vi "Save to Excel (SubVI).vi"(0 "File Path Input":path, 1 "Save (Enable/Signal)":bool, 2 "Save Interval (s)":dbl=1.0, 3 "Title Block Array":string[](array[string]), 4 "Column Header Array":string[](array[string]), 5 "Data Array (Row)":string[](array[string]), 7 "File Configuration":T1={"Row Limit"=65500, "Default File Name"="Data", "New File Daily?"=TRUE, "Manual Save Interval?"=FALSE}, 9 "Change Save Location?":bool, 11 "Reset Elapsed Time":bool caption="Reset Elapsed Time?", 13 "Comments":string) -> (14 "File Path Output":path, 15 "Save Indicator":bool, 16 "# of Rows Saved":i32, 17 "Elapsed Time":string="00:00:00", 19 "Error Output":errorcluster)   [LabVIEW 2009]
panel:
  # "SAVE TO EXCEL SUBVI\nSave 1D Array (Row) to File"
  # "Created by Blake Otting 3/7/2007\nLast Updated 4/8/2010"
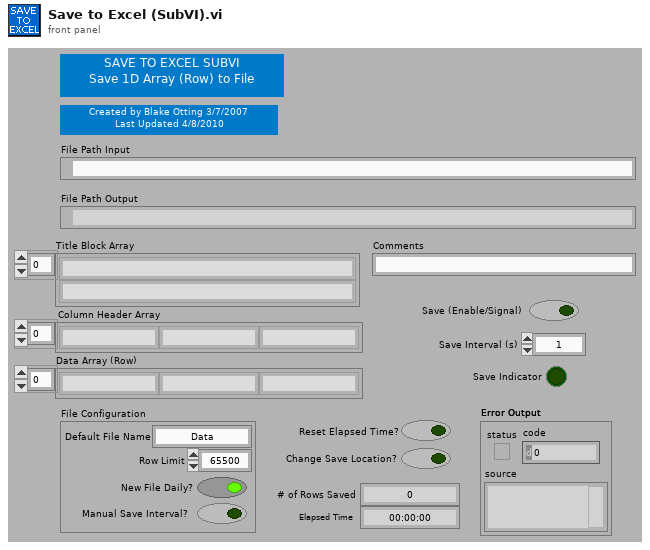
[diagram p1: front panel]
types:
  T1 = cluster{"Row Limit":i32, "Default File Name":string, "New File Daily?":bool, "Manual Save Interval?":bool}
  T2 = typedef "LVDateTimeRec.ctl" = cluster{"fractional second":dbl, "second":i32, "minute":i32, "hour":i32, "day of month":i32, "month":i32, "year":i32, "day of week":i32, "day of year":i32, "DST":i32}
  T3 = enum16{"open", "replace", "create", "open or create", "replace or create", "replace or create with confirmation"}
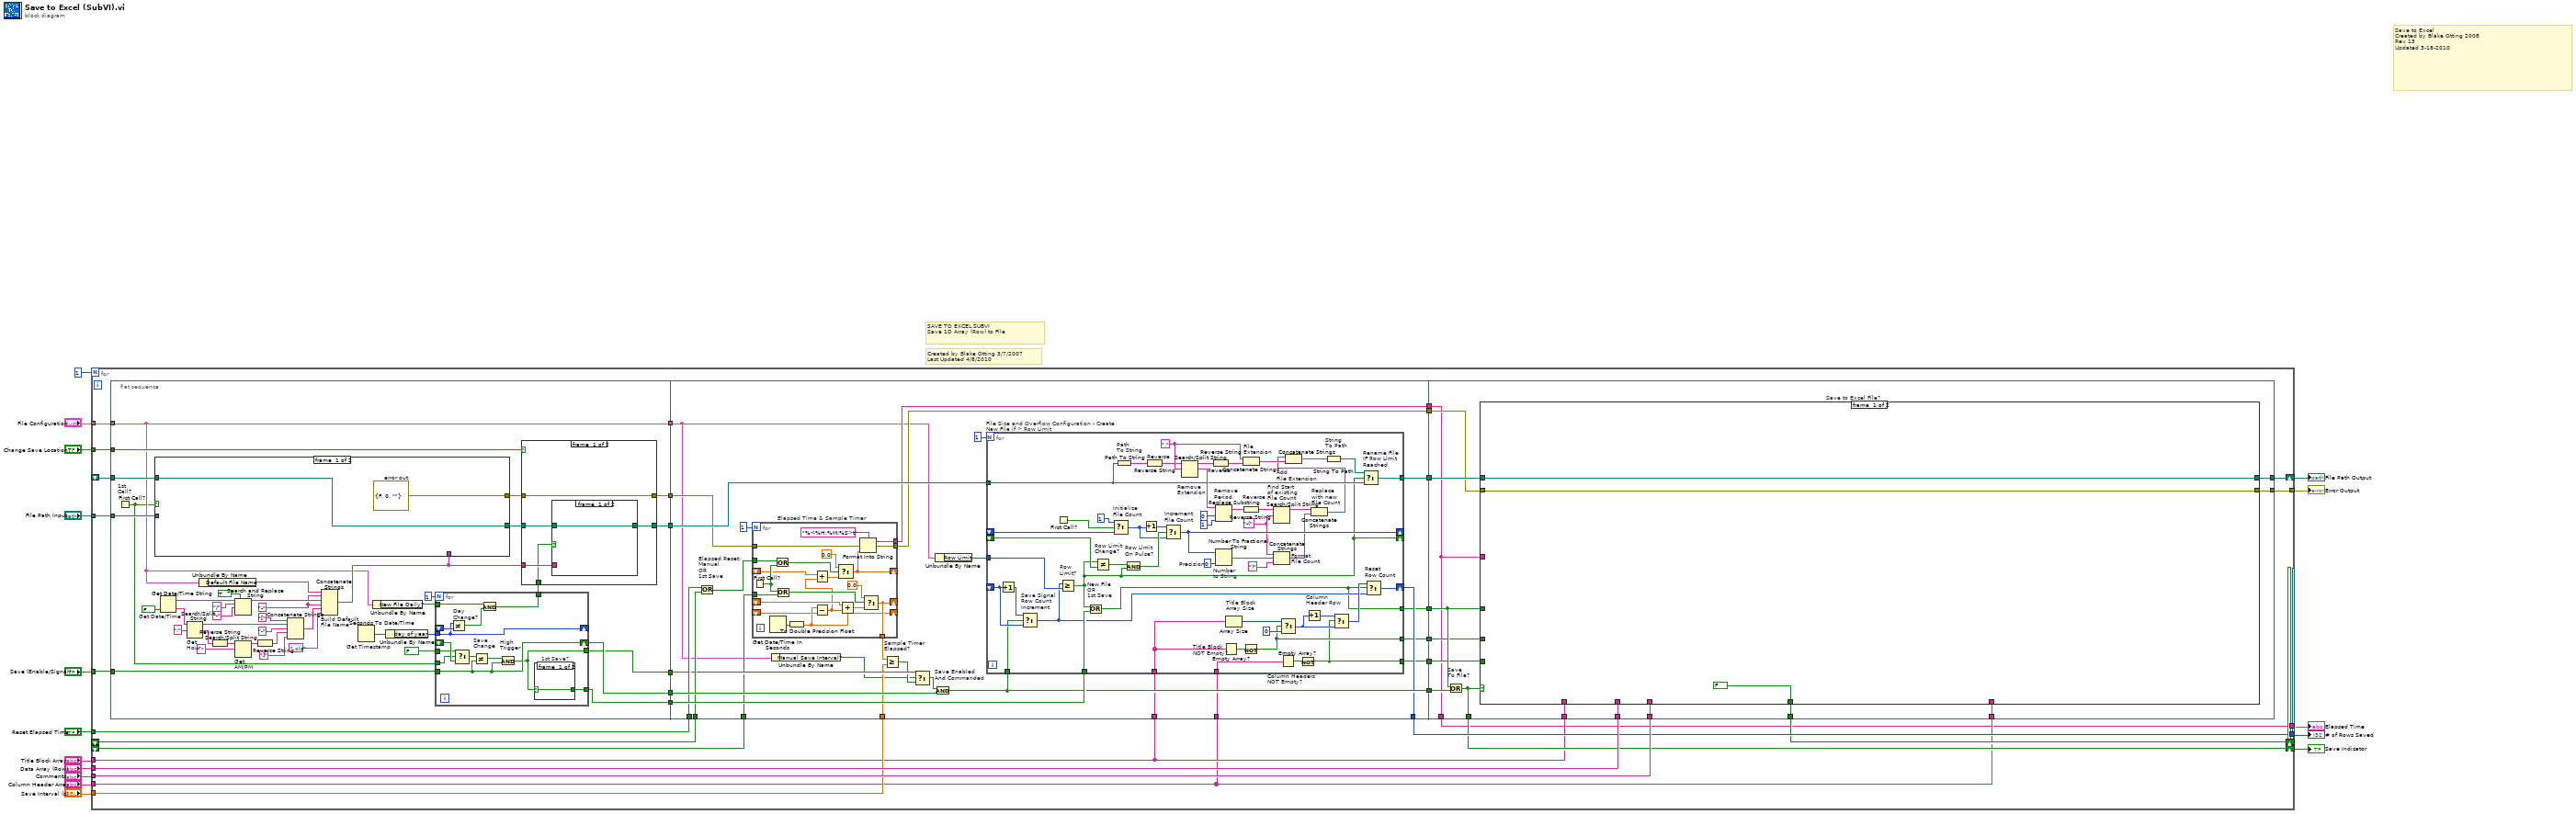
[diagram p0: block diagram]
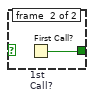
[diagram p2: hidden frame]
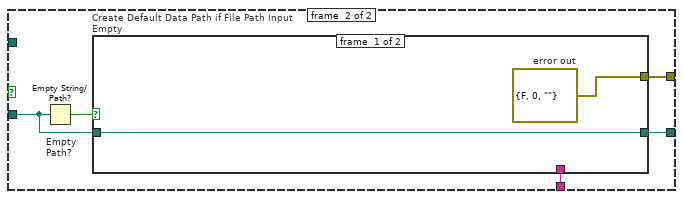
[diagram p3: hidden frame]
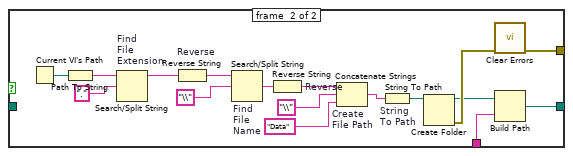
[diagram p4: hidden frame]
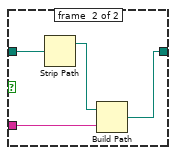
[diagram p5: hidden frame]
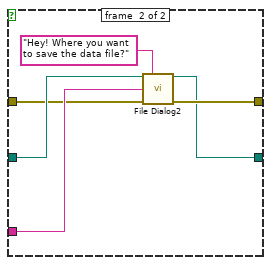
[diagram p6: hidden frame]
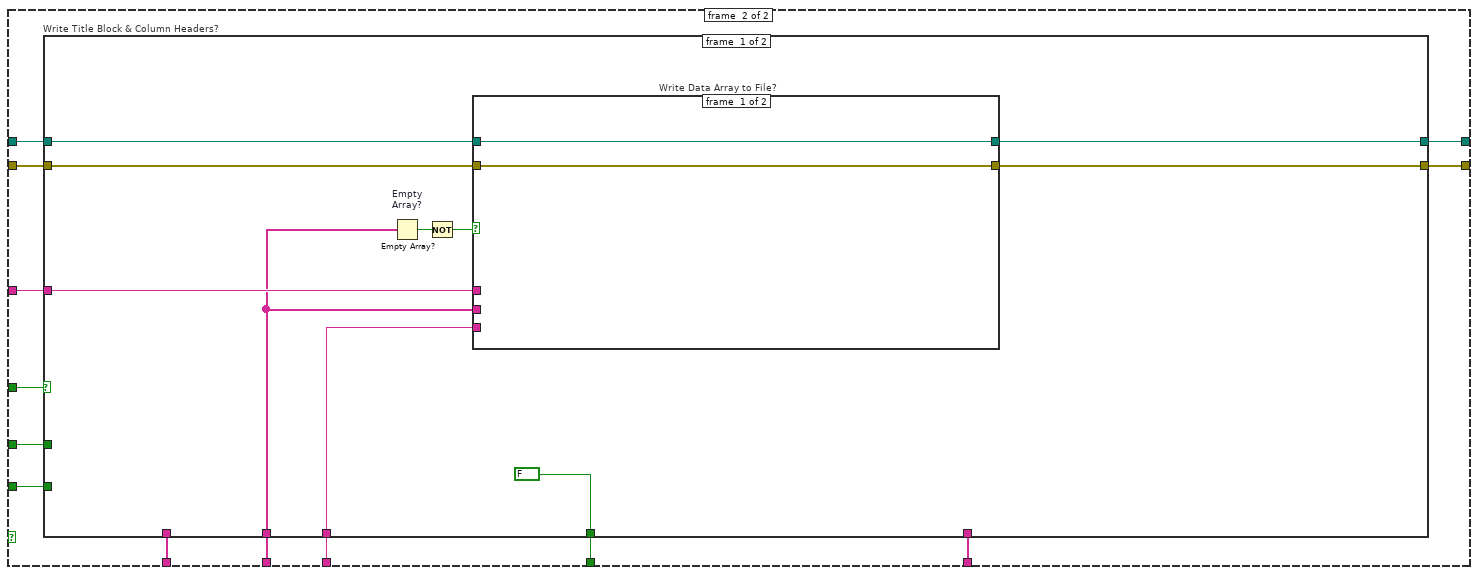
[diagram p7: hidden frame]
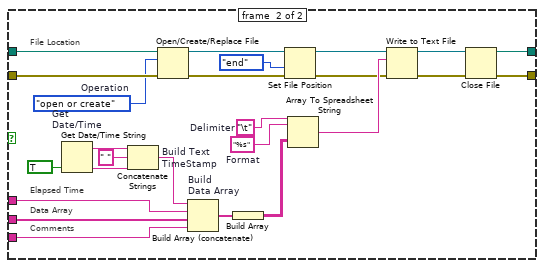
[diagram p8: hidden frame]
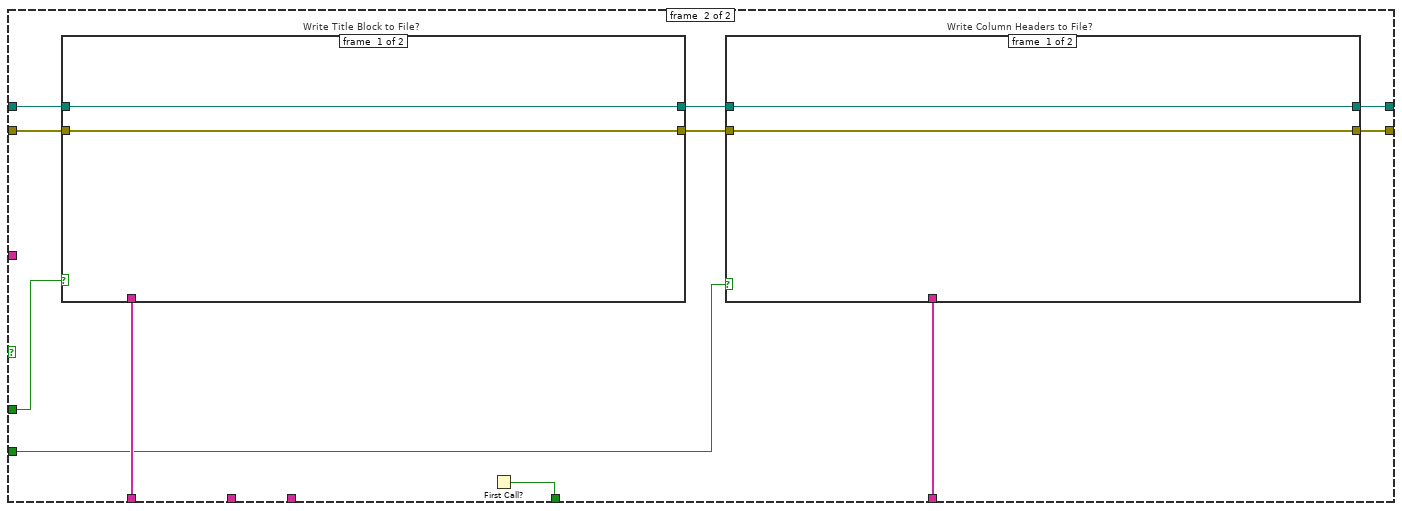
[diagram p9: hidden frame]
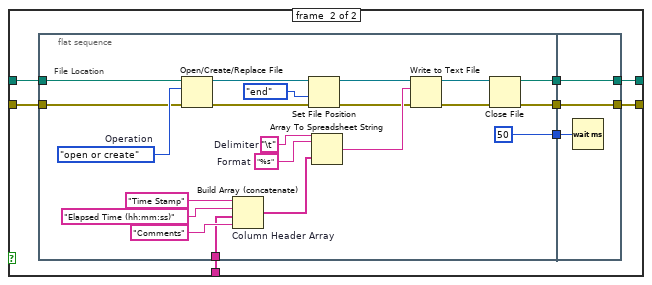
[diagram p10: hidden frame]
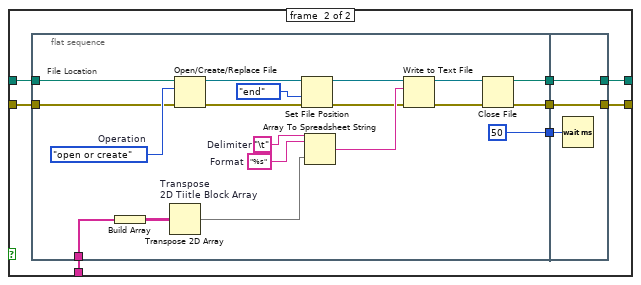
[diagram p11: hidden frame]
diagram:
  # "Created by Blake Otting 3/7/2007\nLast Updated 4/8/2010"
  # "SAVE TO EXCEL SUBVI\nSave 1D Array (Row) to File"
  # "Save to Excel\nCreated by Blake Otting 2008\nRev 13\nUpdated 3-18-2010"
  n1 = for {
    N: 1 -> [_]
    tunnel: "File Path Input" -> [w39]
    tunnel: "Change Save Location?" -> [w48]
    tunnel: "Save (Enable/Signal)" -> [w33]
    tunnel: "Data Array (Row)" -> [w41]
    tunnel: "Column Header Array" -> [w23]
    tunnel: "File Configuration" -> [w29]
    tunnel: "Reset Elapsed Time" -> [w30]
    shift-right: [w35] -> w15
    shift-left: _ -> [w45]
    tunnel: "Save Interval (s)" -> [w34]
    shift-right: [w36] -> _
    shift-left: _ -> [w31]
    tunnel: "Title Block Array" -> [w25]
    tunnel: "Comments" -> [w40]
    shift-right: [w42] -> w13
    shift-left: _ -> [w38]
    tunnel: [w19] -> w14
    tunnel: [w37] -> w16
    tunnel: [w26] -> w12
    n2 = flat-sequence {
      tunnel: w38 -> [w59]
      tunnel: w39 -> [w58]
      tunnel: w48 -> [w51]
      tunnel: w29 -> [w50]
      tunnel: [w53] -> w47
      tunnel: [w55] -> w46
      tunnel: w33 -> [w57]
      tunnel: [w56] -> w32
      tunnel: [w52] -> w28
      tunnel: [w50] -> w18
      tunnel: [w54] -> w17
      tunnel: [w173] -> w44
      tunnel: [w150] -> w43
      tunnel: w45 -> [w155]
      tunnel: w46 -> [w153]
      tunnel: w47 -> [w174]
      tunnel: [w165] -> w37
      tunnel: w34 -> [w152]
      tunnel: w32 -> [w171]
      tunnel: w31 -> [w168]
      tunnel: w30 -> [w167]
      tunnel: w28 -> [w166]
      tunnel: [w156] -> w27
      tunnel: w25 -> [w164]
      tunnel: [w162] -> w24
      tunnel: w23 -> [w161]
      tunnel: [w160] -> w22
      tunnel: [w159] -> w21
      tunnel: [w149] -> w20
      tunnel: w18 -> [w148]
      tunnel: w17 -> [w163]
      tunnel: w44 -> [w261]
      tunnel: w43 -> [w247]
      tunnel: [w259] -> w42
      tunnel: w25 -> [w258]
      tunnel: w41 -> [w257]
      tunnel: w23 -> [w256]
      tunnel: w40 -> [w255]
      tunnel: [w254] -> w35
      tunnel: [w253] -> w36
      tunnel: w27 -> [w252]
      tunnel: [w251] -> w26
      tunnel: w24 -> [w260]
      tunnel: w22 -> [w250]
      tunnel: w21 -> [w249]
      tunnel: w20 -> [w248]
      tunnel: [w247] -> w19
      frame #0 {
        w70 = "-" ("string")
        n3 = First Call? "1st\nCall?"() -> (First Call?: T/F=w49:bool)
        n4 = Get Date/Time String "Get Date/Time"(want seconds? (F)=FALSE) -> (date string=w65:string, time string=w64:string)  [unwired: 2 out]
        n5 = Search/Split String "Get\nHour"(string=w64, search string/char (-)=":" ("search string")) -> (substring before match=w75:string, match + rest of string=w72:string)  [unwired: 2 out]
        n6 = Unbundle By Name(w50) -> ("Default File Name"=w81:string)
        n7 = Reverse String(1:w72) -> (0:w73:string)
        n8 = Search and Replace String(replace all?=TRUE ("replace all? (F)"), input string=w65, search string="/", replace string="-" ("replace string (\"\")")) -> (result string=w80:string)  [unwired: 1 in, 6 out]
        n9 = Search/Split String "Get\nAM/PM"(string=w73, search string/char (-)=" ") -> (substring before match=w74:string)  [unwired: 3 out]
        n10 = Reverse String(1:w74) -> (0:w76:string)
        n11 = Concatenate Strings ("Build\nHour String")("[" ("string"), w75, "-" ("search string/char (-)"), w76, "]" ("string")) -> (w67:string)
        n12 = Concatenate Strings "Build Default\nFile Name"(w81, w70, w80, w70, w67, ".xls" ("string")) -> (w89:string)
        n13 = case shown="True" w49 {
          tunnel: w58 -> [_ w110]
          tunnel: [w106 w109] -> w60
          tunnel: w89 -> [_ w108]
          tunnel: [w105 w107] -> w82
          tunnel: w59 -> [w106 _]
          frame #0 {
            w105 = errorcluster {"status"=FALSE, "code"=0, "source"=""}  # error out
          }
          frame #1 {
            n14 = Empty String/Path? "Empty\nPath?"(string/path=w110) -> (empty?=w111:bool)
            n15 = case "Create Default Data Path if File Path Input Empty" shown="True" w111 {
              tunnel: [w113 w116] -> w109
              tunnel: w110 -> [w113 _]
              tunnel: w108 -> [_ w115]
              tunnel: [w112 w114] -> w107
              frame #0 {
                w112 = errorcluster {"status"=FALSE, "code"=0, "source"=""}  # error out
              }
              frame #1 {
                n16 = Current VI's Path() -> (path=w122:path)
                n17 = Path To String(path=w122) -> (string=w128:string)
                n18 = Search/Split String "Find\nFile \nExtension"(string=w128, search string/char (-)=".") -> (substring before match=w127:string)  [unwired: 1 in, 2 out]
                n19 = Reverse String "Reverse"(1:w127) -> (0:w126:string)
                n20 = Search/Split String "Find\nFile \nName"(string=w126, search string/char (-)="\\") -> (match + rest of string=w124:string)  [unwired: 1 in, 2 out]
                n21 = Reverse String "Reverse"(1:w124) -> (0:w123:string)
                n22 = Concatenate Strings "Create\nFile Path"(w123, "\\", "Data") -> (w130:string)
                n23 = String To Path "String\nTo Path"(string=w130) -> (path=w120:path)
                n24 = Create Folder(path (use dialog)=w120) -> (created path=w117:path, error out=w119:errorcluster)  [unwired: 2 in, 1 out]
                n25 = call <vilib>:"Clear Errors.vi"("error in (no error)"=w119) -> ("error out"=w114:errorcluster)  [unwired: 6 in]
                n26 = Build Path(base path=w117, name or relative path=w115) -> (appended path=w116:path)
              }
            }
          }
        }
        n27 = Seconds To Date/Time "Get Timestamp"() -> (date time rec=w87:T2)  [unwired: 2 out]
        n28 = Unbundle By Name(w50) -> ("New File Daily?"=w83:bool)
        n29 = Unbundle By Name(w87) -> ("day of year"=w84:i32)
        n30 = for {
          N: 1 -> [_]
          tunnel: w57 -> [w101]
          shift-right: [w101] -> w56
          shift-left: _ -> [w95]
          tunnel: w84 -> [w99]
          shift-right: [w99] -> _
          shift-left: _ -> [w100]
          tunnel: w83 -> [w97]
          tunnel: [w96] -> w86
          tunnel: [w93] -> w53
          tunnel: [w92] -> w52
          tunnel: w49 -> [w91]
          tunnel: FALSE -> [w90]
          n31 = Not Equal? "Day\nChange?"(x=w99, y=w100) -> (x != y?=w98:bool)
          n32 = Select(t=w90, s=w91, f=w95) -> (s? t:f=w94:bool)
          n33 = Not Equal? "Save\nChange"(x=w94, y=w101) -> (x != y?=w102:bool)
          n34 = And(x=w97, y=w98) -> (x .and. y?=w96:bool)
          n35 = And "High\nTrigger"(x=w102, y=w101) -> (x .and. y?=w92:bool)
          n36 = case "1st Save?" shown="True" w92 {
            selector: w92 -> [w103 _]
            tunnel: [w103 w104] -> w93
            frame #0 {
            }
            frame #1 {
              n37 = First Call? "1st\nCall?"() -> (First Call?: T/F=w104:bool)
            }
          }
        }
        n38 = case shown="False" w51 {
          tunnel: w60 -> [w134 w146]
          tunnel: w89 -> [w133 w144]
          tunnel: w82 -> [w135 w143]
          tunnel: [w135 w142] -> w55
          tunnel: w86 -> [w132 _]
          tunnel: [w131 w141] -> w54
          frame #0 {
            n39 = case shown="True" w132 {
              tunnel: w134 -> [w136 w140]
              tunnel: w133 -> [_ w138]
              tunnel: [w136 w137] -> w131
              frame #0 {
              }
              frame #1 {
                n40 = Strip Path(path=w140) -> (stripped path=w139:path)  [unwired: 1 out]
                n41 = Build Path(base path=w139, name or relative path=w138) -> (appended path=w137:path)
              }
            }
          }
          frame #1 {
            n42 = call "File Dialog2"("start path"=w146, "prompt"="Hey! Where you want to save the data file?", "default name"=w144, "error in"=w143) -> ("selected path"=w141:path, "error out"=w142:errorcluster)  [unwired: 3 in, 7 out]
          }
        }
      }
      frame #1 {
        n43 = Or "Elapsed Reset:\nManual\nOR\n1st Save"(x=w167, y=w168) -> (x .or. y?=w151:bool)
        n44 = for "Elapsed Time & Sample Timer" {
          N: 1 -> [_]
          shift-right: [w192] -> _
          shift-left: _ -> [w195]
          shift-right: [w184] -> _
          shift-left: _ -> [w194]
          tunnel: [w192] -> w157
          tunnel: w155 -> [w188]
          tunnel: w151 -> [w186]
          shift-right: [w179] -> _
          shift-left: _ -> [w183]
          tunnel: [w177] -> w150
          tunnel: [w176] -> w156
          tunnel: w153 -> [w175]
          n45 = First Call?() -> (First Call?: T/F=w187:bool)
          n46 = Get Date/Time In Seconds() -> (seconds since 1Jan1904=w193:timestamp)
          n47 = Or(x=w186, y=w187) -> (x .or. y?=w181:bool)
          n48 = Or(x=w187, y=w188) -> (x .or. y?=w189:bool)
          n49 = To Double Precision Float(number=w193) -> (double precision float=w184:dbl)
          n50 = Subtract(x=w184, y=w194) -> (x-y=w178:dbl)
          n51 = Add(x=w183, y=w178) -> (x+y=w185:dbl)
          n52 = Select(t=0.0, s=w181, f=w185) -> (s? t:f=w179:dbl)
          n53 = Add(x=w195, y=w178) -> (x+y=w191:dbl)
          n54 = Format Into String(format string="%<%H:%M:%S>t", error in=w175, w179) -> (resulting string=w177:string, error out=w176:errorcluster)  [unwired: 1 in]
          n55 = Select(t=0.0, s=w189, f=w191) -> (s? t:f=w192:dbl)
        }
        n56 = Unbundle By Name(w148) -> ("Manual Save Interval?"=w147:bool)
        n57 = Greater Or Equal? "Sample Timer\nElapsed?"(x=w157, y=w152) -> (x >= y?=w154:bool)
        n58 = Select(t=w166, s=w147, f=w154) -> (s? t:f=w172:bool)
        n59 = And "Save Enabled\nAnd Commanded"(x=w172, y=w171) -> (x .and. y?=w173:bool)
        n60 = Unbundle By Name(w148) -> ("Row Limit"=w170:i32)
        n61 = for "File Size and Overflow Configuration - Create New File if > Row Limit" {
          N: 1 -> [_]
          tunnel: w174 -> [w244]
          tunnel: w173 -> [w243]
          shift-right: [w241] -> w165
          shift-left: _ -> [w245]
          tunnel: w170 -> [w242]
          shift-right: [w209] -> _
          shift-left: _ -> [w240]
          tunnel: w164 -> [w205]
          shift-right: [w234] -> _
          shift-left: _ -> [w212]
          tunnel: w163 -> [w223]
          tunnel: [w215] -> w162
          tunnel: w161 -> [w207]
          tunnel: [w199] -> w159
          tunnel: [w198] -> w149
          tunnel: [w196] -> w160
          w232 = "." ("search string/char (-)")
          w216 = "-("
          w238 = i16 0  # Precision
          n62 = Increment(x=w245) -> (x+1=w246:i32)
          n63 = Select "Save Signal\nRow Count\nIncrement"(t=w246, s=w243, f=w245) -> (s? t:f=w197:i32)
          n64 = First Call?() -> (First Call?: T/F=w213:bool)
          n65 = Greater Or Equal? "Row\nLimit?"(x=w197, y=w242) -> (x >= y?=w209:bool)
          n66 = Or "New File\nOR\n1st Save"(x=w209, y=w244) -> (x .or. y?=w196:bool)
          n67 = Not Equal? "Row Limit\nChange?"(x=w209, y=w240) -> (x != y?=w235:bool)
          n68 = Select "Initialize\nFile Count"(t=i16 1, s=w213, f=w212) -> (s? t:f=w211:i16)
          n69 = Path To String "Path\nTo String"(path=w223) -> (string=w225:string)
          n70 = And "Row Limit\nOn Pulse?"(x=w235, y=w209) -> (x .and. y?=w239:bool)
          n71 = Increment(x=w211) -> (x+1=w236:i16)
          n72 = Reverse String "Reverse"(1:w225) -> (0:w226:string)
          n73 = Select "Increment\nFile Count"(t=w236, s=w239, f=w211) -> (s? t:f=w234:i16)
          n74 = Search/Split String "Remove\nExtension"(string=w226, search string/char (-)=w232) -> (substring before match=w227:string, match + rest of string=w228:string)  [unwired: 2 out]
          n75 = Reverse String "Reverse"(1:w227) -> (0:w224:string)
          n76 = Replace Substring "Remove\nPeriod"(2:1 ("length (len. of substring)"), 3:0 ("offset (0)"), 5:w228) -> (1:w229:string)  [unwired: 2 out]
          n77 = Number To Fractional String "Number\nto String"(number=w234, precision (6)=w238) -> (F-format string=w237:string)  [unwired: 2 in]
          n78 = Empty Array? "Title Block\nNOT Empty?"(array=w205) -> (empty?=w206:bool)
          n79 = Array Size "Title Block\nArray Size"(array=w205) -> (size(s)=w204:i32)
          n80 = Reverse String "Reverse"(1:w229) -> (0:w221:string)
          n81 = Not(x=w206) -> (.not. x?=w199:bool)
          n82 = Concatenate Strings "File\nExtension"(w232, w224) -> (w218:string)
          n83 = Search/Split String "Find Start\nof existing\nFile Count"(string=w221, search string/char (-)=w216) -> (substring before match=w220:string)  [unwired: 1 in, 2 out]
          n84 = Concatenate Strings "Format\nFile Count"(w216, w237, ")") -> (w219:string)
          n85 = Empty Array? "Column Headers\nNOT Empty?"(array=w207) -> (empty?=w208:bool)
          n86 = Select(t=w204, s=w199, f=0 ("t")) -> (s? t:f=w202:i32)
          n87 = Not(x=w208) -> (.not. x?=w198:bool)
          n88 = Increment "Column\nHeader Row"(x=w202) -> (x+1=w201:i32)
          n89 = Concatenate Strings "Replace\nwith new\nFile Count"(w220, w219) -> (w210:string)
          n90 = Concatenate Strings "Add\nFile Extension"(w210, w218) -> (w217:string)
          n91 = String To Path "String\nTo Path"(string=w217) -> (path=w233:path)
          n92 = Select(t=w201, s=w198, f=w202) -> (s? t:f=w200:i32)
          n93 = Select "Rename File\nIF Row Limit\nReached"(t=w233, s=w209, f=w223) -> (s? t:f=w215:path)
          n94 = Select "Reset\nRow Count"(t=w200, s=w196, f=w197) -> (s? t:f=w241:i32)
        }
      }
      frame #2 {
        n95 = Or "Save\nTo File?"(x=w250, y=w261) -> (x .or. y?=w254:bool)
        n96 = case "Save to Excel File?" shown="True" w254 {
          tunnel: [w264 w277] -> w259
          tunnel: w260 -> [w264 w276]
          tunnel: w250 -> [_ w275]
          tunnel: [FALSE ("First Call?: T/F") w274] -> w253
          tunnel: w247 -> [_ w273]
          tunnel: w258 -> [_ w270]
          tunnel: w257 -> [_ w272]
          tunnel: w256 -> [_ w271]
          tunnel: w255 -> [_ w269]
          tunnel: w252 -> [w262 w268]
          tunnel: [w262 w267] -> w251
          tunnel: w249 -> [_ w266]
          tunnel: w248 -> [_ w265]
          frame #0 {
          }
          frame #1 {
            n97 = case "Write Title Block & Column Headers?" shown="True" w275 {
              tunnel: [w285 w320] -> w277
              tunnel: w276 -> [w286 w324]
              tunnel: w270 -> [_ w318]
              tunnel: w271 -> [_ w317]
              tunnel: w273 -> [w284 _]
              tunnel: [FALSE ("First Call?: T/F") w325] -> w274
              tunnel: w269 -> [w282 _]
              tunnel: w272 -> [w279 _]
              tunnel: w268 -> [w283 w321]
              tunnel: [w281 w319] -> w267
              tunnel: w266 -> [_ w316]
              tunnel: w265 -> [_ w315]
              frame #0 {
                n98 = Empty Array? "Empty\nArray?"(array=w279) -> (empty?=w280:bool)
                n99 = Not(x=w280) -> (.not. x?=w278:bool)
                n100 = case "Write Data Array to File?" shown="True" w278 {
                  tunnel: w286 -> [w289 w314]
                  tunnel: [w289 w313] -> w285
                  tunnel: w279 -> [_ w312]
                  tunnel: w284 -> [_ w311]
                  tunnel: w283 -> [w288 w310]
                  tunnel: w282 -> [_ w309]
                  tunnel: [w288 w308] -> w281
                  frame #0 {
                  }
                  frame #1 {
                    w297 = "\t"  # Delimiter
                    w296 = "%s"  # Format
                    w304 = T3."open or create"  # Operation
                    # "Comments"
                    # "Data Array"
                    # "Elapsed Time"
                    # "File Location"
                    n101 = Get Date/Time String "Get \nDate/Time"(want seconds? (F)=TRUE) -> (date string=w299:string, time string=w302:string)  [unwired: 2 out]
                    n102 = Concatenate Strings "Build Text\nTimeStamp"(w299, " " ("string"), w302) -> (w303:string)
                    n103 = Open/Create/Replace File(file path (use dialog)=w314, error in=w310, operation (0:open)=w304) -> (refnum out=w290:refnum<file>, error out=w291:errorcluster)  [unwired: 3 in, 1 out]
                    n104 = Build Array (concatenate) "Build\nData Array"(w303, w311, w312, w309) -> (w306:string[])
                    n105 = Build Array(w306) -> (w307:string[][])
                    n106 = Set File Position(refnum=w290, from (0:start)=enum16{"start", "end", "current"}."end", error in=w291) -> (refnum out=w292:refnum<file>, error out=w293:errorcluster)  [unwired: 1 in]
                    n107 = Array To Spreadsheet String(delimiter (Tab)=w297, array=w307, 3:w296) -> (spreadsheet string=w298:string)
                    n108 = Write to Text File(file (use dialog)=w292, text=w298, error in=w293) -> (refnum out=w294:refnum<file>, error out=w295:errorcluster)  [unwired: 1 in, 1 out]
                    n109 = Close File(refnum=w294, error in=w295) -> (path=w313:path, error out=w308:errorcluster)
                  }
                }
              }
              frame #1 {
                n110 = case "Write Title Block to File?" shown="True" w316 {
                  tunnel: w324 -> [w360 w369]
                  tunnel: w318 -> [_ w368]
                  tunnel: [w361 w367] -> w322
                  tunnel: [w360 w366] -> w323
                  tunnel: w321 -> [w361 w365]
                  frame #0 {
                  }
                  frame #1 {
                    n111 = flat-sequence "Write to Excel File" {
                      tunnel: w368 -> [w372]
                      tunnel: w369 -> [w377]
                      tunnel: w365 -> [w371]
                      tunnel: [w376] -> w364
                      tunnel: [w375] -> w363
                      tunnel: [u32 50 ("milliseconds to wait")] -> w362
                      tunnel: [w390] -> w367
                      tunnel: [w391] -> w366
                      tunnel: w364 -> [w391]
                      tunnel: w363 -> [w390]
                      tunnel: w362 -> [w389]
                      frame #0 {
                        w385 = "\t"  # Delimiter
                        w384 = "%s"  # Format
                        w387 = T3."open or create"  # Operation
                        # "File Location"
                        n112 = Build Array(w372) -> (w374:string[][])
                        n113 = Transpose 2D Array "Transpose\n2D Tiitle Block Array"(2D array=w374) -> (transposed array=w373:string[][])
                        n114 = Open/Create/Replace File(file path (use dialog)=w377, error in=w371, operation (0:open)=w387) -> (refnum out=w378:refnum<file>, error out=w379:errorcluster)  [unwired: 3 in, 1 out]
                        n115 = Set File Position(refnum=w378, from (0:start)=enum16{"start", "end", "current"}."end", error in=w379) -> (refnum out=w380:refnum<file>, error out=w381:errorcluster)  [unwired: 1 in]
                        n116 = Array To Spreadsheet String(delimiter (Tab)=w385, array=w373, 3:w384) -> (spreadsheet string=w386:string)
                        n117 = Write to Text File(file (use dialog)=w380, text=w386, error in=w381) -> (refnum out=w382:refnum<file>, error out=w383:errorcluster)  [unwired: 1 in, 1 out]
                        n118 = Close File(refnum=w382, error in=w383) -> (path=w376:path, error out=w375:errorcluster)
                      }
                      frame #1 {
                        n119 = Wait (ms)(milliseconds to wait=w389) -> ()  [unwired: 1 out]
                      }
                    }
                  }
                }
                n120 = First Call?() -> (First Call?: T/F=w325:bool)
                n121 = case "Write Column Headers to File?" shown="True" w315 {
                  tunnel: w323 -> [w326 w335]
                  tunnel: [w327 w334] -> w319
                  tunnel: w322 -> [w327 w333]
                  tunnel: [w326 w332] -> w320
                  tunnel: w317 -> [_ w331]
                  frame #0 {
                  }
                  frame #1 {
                    n122 = flat-sequence "Write to Excel File" {
                      tunnel: w335 -> [w345]
                      tunnel: w333 -> [w342]
                      tunnel: w331 -> [w337]
                      tunnel: [w344] -> w330
                      tunnel: [w343] -> w329
                      tunnel: [u32 50 ("milliseconds to wait")] -> w328
                      tunnel: [w358] -> w334
                      tunnel: [w359] -> w332
                      tunnel: w330 -> [w359]
                      tunnel: w329 -> [w358]
                      tunnel: w328 -> [w357]
                      frame #0 {
                        w353 = "\t"  # Delimiter
                        w352 = "%s"  # Format
                        w355 = T3."open or create"  # Operation
                        # "File Location"
                        n123 = Open/Create/Replace File(file path (use dialog)=w345, error in=w342, operation (0:open)=w355) -> (refnum out=w346:refnum<file>, error out=w347:errorcluster)  [unwired: 3 in, 1 out]
                        n124 = Build Array (concatenate) "Column Header Array"("Time Stamp", "Elapsed Time (hh:mm:ss)", w337, "Comments") -> (w338:string[])
                        n125 = Set File Position(refnum=w346, from (0:start)=enum16{"start", "end", "current"}."end", error in=w347) -> (refnum out=w348:refnum<file>, error out=w349:errorcluster)  [unwired: 1 in]
                        n126 = Array To Spreadsheet String(delimiter (Tab)=w353, array=w338, 3:w352) -> (spreadsheet string=w354:string)
                        n127 = Write to Text File(file (use dialog)=w348, text=w354, error in=w349) -> (refnum out=w350:refnum<file>, error out=w351:errorcluster)  [unwired: 1 in, 1 out]
                        n128 = Close File(refnum=w350, error in=w351) -> (path=w344:path, error out=w343:errorcluster)
                      }
                      frame #1 {
                        n129 = Wait (ms)(milliseconds to wait=w357) -> ()  [unwired: 1 out]
                      }
                    }
                  }
                }
              }
            }
          }
        }
      }
    }
  }
  "# of Rows Saved" <- w16
  "Save Indicator" <- w15
  "File Path Output" <- w13
  "Error Output" <- w12
  "Elapsed Time" <- w14
